vi "LoadExporterConfigurationPage.vi"(8 "error in (no error)":errorcluster, 9 "Selection":string, 11 "UIManager in":refnum<class "UIManager.lvclass">) -> (0 "error out":errorcluster, 1 "References":T1, 3 "UIManager out":refnum<class "UIManager.lvclass">)   [LabVIEW 2020, in "UserInterface.lvlib" / "UIManager.lvclass"]
uses:
  UIManager.lvclass
  Private/subReferenceData.ctl
  ExtensionInterfaces/IConfigurationPage/Event_Stop.ctl
  ExtensionInterfaces/IConfigurationPage/Event_Parameters.ctl
  UIManager.lvclass/UIManager.ctl
  ExtensionInterfaces/IExporter/IExporter.lvclass
  ExtensionInterfaces/IConfigurationPage/IConfigurationPage.lvclass
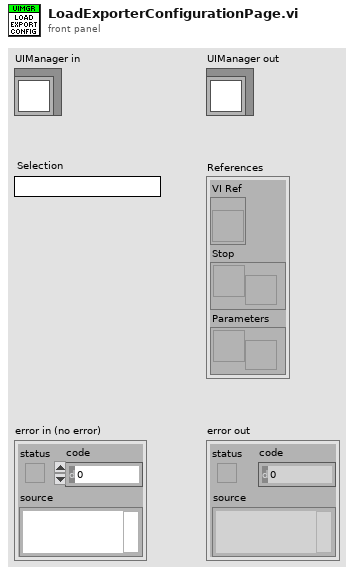
[diagram p1: front panel]
types:
  T1 = typedef "UserInterface.lvlib/UIManager.lvclass/subReferenceData.ctl" = cluster{"VI Ref":refnum<vi>, "Stop":refnum<user-event>, "Parameters":refnum<user-event>}
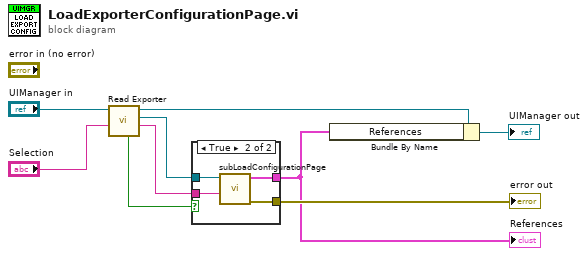
[diagram p0: block diagram]
diagram:
  n1 = call-dynamic "Read Exporter.vi"("Selection"="Selection", "UIManager in"="UIManager in") -> ("Parameters"=w2:string, "IExporter.lvclass"=w4:refnum<class "IExporter.lvclass">, "UIManager out"=w1:refnum<class "UIManager.lvclass">, "found?"=w3:bool)  [unwired: 6 in]
  n2 = case shown="True" w3 {
    tunnel: w4 -> [_ w13]
    tunnel: [_ w12] -> w9
    tunnel: [_ w11] -> w8
    tunnel: w2 -> [_ w10]
    frame False {
    }
    frame True {
      n3 = call "subLoadConfigurationPage.vi"("Parameters"=w10, "Interface in"=w13) -> ("error out"=w12:errorcluster, "References"=w11:T1)  [unwired: 8 in]
    }
  }
  "error out" <- w9
  "References" <- w8
  n4 = Bundle By Name(cluster=w1, "References"=w8) -> (→"UIManager out":refnum<class "UIManager.lvclass">)
